vi "BuildHWI.vi"(8 "error in (no error)":errorcluster, 10 "Master Device in":refnum<class "Master Device.lvclass">, 11 "Advanced_DMD in":refnum<class "Advanced_DMD.lvclass">) -> (0 "error out":errorcluster, 2 "Master Device out":refnum<class "Master Device.lvclass">, 3 "Advanced_DMD out":refnum<class "Advanced_DMD.lvclass">)   [LabVIEW 2013, in "Advanced_DMD.lvclass"]
doc: "The previous subVI Prune.vi took the \"prepared\" private data and removed unnecessary points. Here in BuildHWI, one should turn the \"prepared\" data into a HWI that can be programmed to the physical device.\n (1) Flatten the data structure and put in normal time order"
uses:
  Advanced_DMD.lvclass
  Master Device/Master Device.lvclass
  Advanced_DMD.lvclass/Advanced_DMD.ctl
panel:
  out "appended path":path
  out "matlab command":string
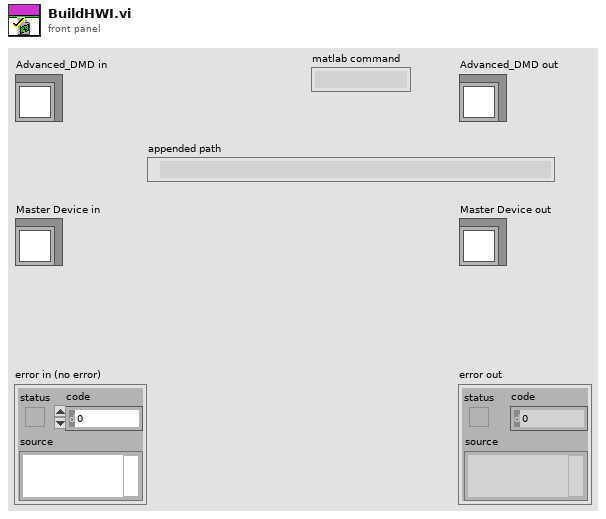
[diagram p1: front panel]
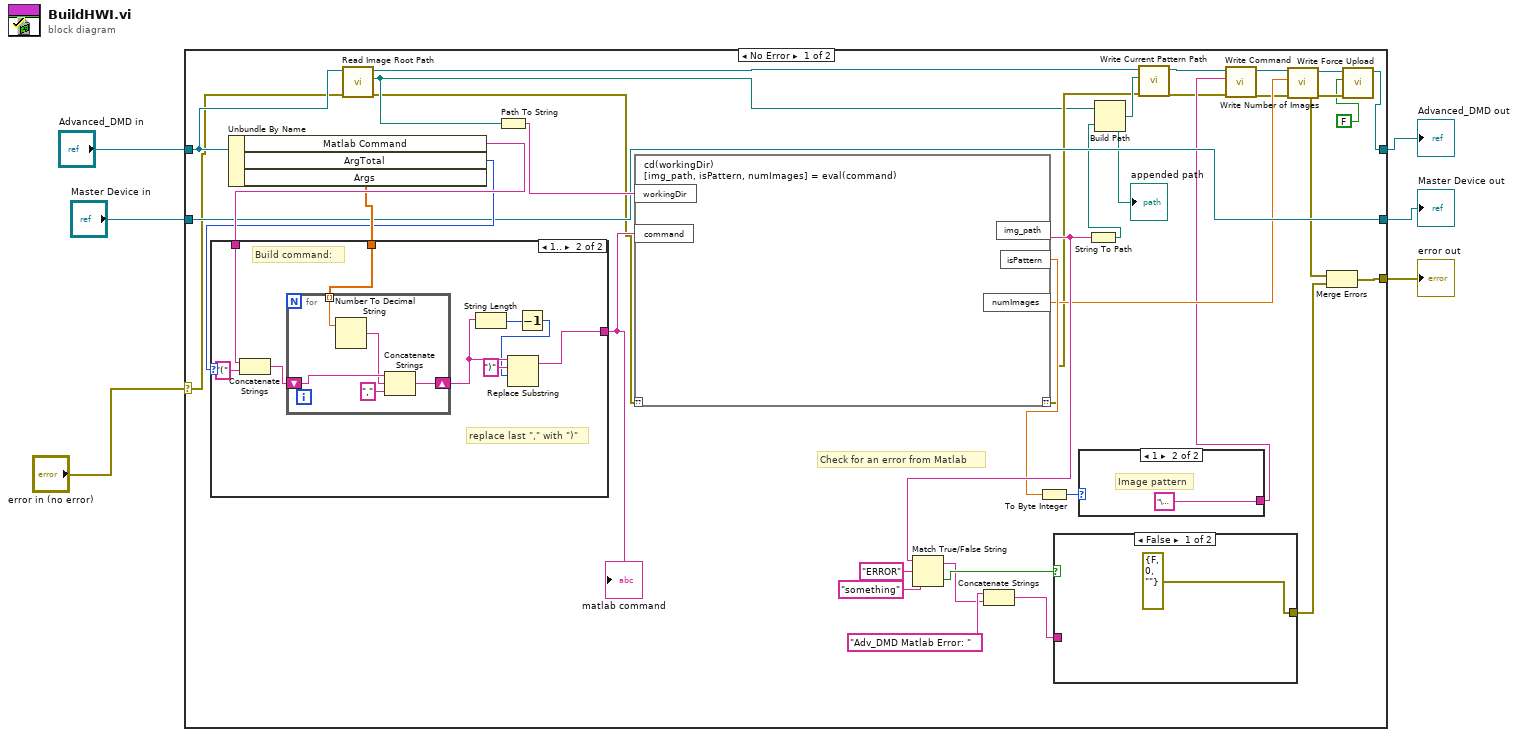
[diagram p0: block diagram]
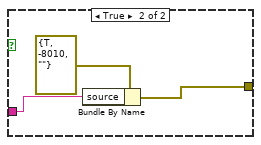
[diagram p2: hidden frame]
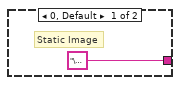
[diagram p3: hidden frame]
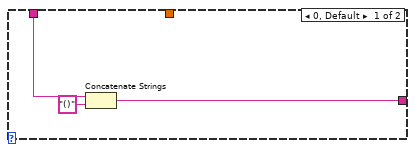
[diagram p4: hidden frame]
diagram:
  n1 = case shown="No Error" "error in (no error)" {
    selector: "error in (no error)" -> [w10 w66]
    tunnel: "Advanced_DMD in" -> [w11 w68]
    tunnel: [w20 w68] -> w4
    tunnel: [w37 w67] -> w3
    tunnel: "Master Device in" -> [w37 w67]
    tunnel: [w28 w66] -> w1
    frame No Error {
      # "Check for an error from Matlab"
      n2 = Unbundle By Name(w11) -> ("Matlab Command"=w41:string, "ArgTotal"=w39:u8, "Args"=w40:dbl[])
      n3 = case shown="1.." w39 {
        tunnel: w41 -> [w51 w59]
        tunnel: w40 -> [_ w57]
        tunnel: [w49 w52] -> w38
        frame 0, Default {
          n4 = Concatenate Strings(w51, "()" ("string")) -> (w49:string)
        }
        frame 1.. {
          # "replace last \",\" with \")\""
          # "Build command:"
          n5 = Concatenate Strings(w59, "(" ("string")) -> (w58:string)
          n6 = for {
            shift-right: [w61] -> w55
            shift-left: w58 -> [w65]
            tunnel: w57 -> [w64] mode=indexing
            n7 = Number To Decimal String(number=w64) -> (decimal integer string=w63:string)  [unwired: 1 in]
            n8 = Concatenate Strings(w65, w63, "," ("string")) -> (w61:string)
          }
          n9 = String Length(string=w55) -> (length=w56:i32)
          n10 = Decrement(x=w56) -> (x-1=w53:i32)
          n11 = Replace Substring(3:w53, 4:")" ("substring (\"\")"), 5:w55) -> (1:w52:string)  [unwired: 1 in, 1 out]
        }
      }
      "matlab command" <- w38
      n12 = call-dynamic "Read Image Root Path.vi"("error in (no error)"=w10, "DMD in"=w11) -> ("error out"=w8:errorcluster, "Image Root Path"=w9:path, "DMD out"=w7:refnum<class "Advanced_DMD.lvclass">)  [unwired: 7 in]
      n13 = Path To String(path=w9) -> (string=w42:string)
      n14 = script code="cd(workingDir)\n[img_path, isPattern, numImages] = eval(command)"("??"=w8, "workingDir"=w42, "command"=w38) -> ("??"=w17:errorcluster, "img_path"=w33:string, "isPattern"=w26:dbl, "numImages"=w19:dbl)
      n15 = Match True/False String(2:"something" ("false string"), 3:"ERROR" ("true string"), 4:w33) -> (0:w34:bool, 1:w30:string)
      n16 = Concatenate Strings("Adv_DMD Matlab Error: " ("false string"), w30) -> (w29:string)
      n17 = To Byte Integer(number=w26) -> (8bit integer=w25:i8)
      n18 = case shown="False" w34 {
        tunnel: [errorcluster {"status"=FALSE, "code"=0, "source"=""} ("error out") w44] -> w27
        tunnel: w29 -> [_ w45]
        frame False {
        }
        frame True {
          n19 = Bundle By Name(cluster=errorcluster {"status"=TRUE, "code"=-8010, "source"=""} ("error out"), "source"=w45) -> (w44:errorcluster)
        }
      }
      n20 = case shown="1" w25 {
        tunnel: ["\u0000" "\u0004"] -> w18
        frame 0, Default {
          # "Static Image"
        }
        frame 1 {
          # "Image pattern"
        }
      }
      n21 = String To Path(string=w33) -> (path=w36:path)
      n22 = Build Path(base path=w9, name or relative path=w36) -> (appended path=w24:path)
      "appended path" <- w24
      n23 = call-dynamic "Write Current Pattern Path.vi"("error in (no error)"=w17, "Current Pattern Path"=w24, "DMD in"=w7) -> ("error out"=w16:errorcluster, "DMD out"=w23:refnum<class "Advanced_DMD.lvclass">)  [unwired: 7 in]
      n24 = call-dynamic "Write Command.vi"("error in (no error)"=w16, "Command"=w18, "DMD in"=w23) -> ("error out"=w15:errorcluster, "DMD out"=w22:refnum<class "Advanced_DMD.lvclass">)  [unwired: 7 in]
      n25 = call-dynamic "Write Number of Images.vi"("error in (no error)"=w15, "Number of Images"=w19, "DMD in"=w22) -> ("error out"=w14:errorcluster, "DMD out"=w21:refnum<class "Advanced_DMD.lvclass">)  [unwired: 7 in]
      n26 = call-dynamic "Write Force Upload.vi"("error in (no error)"=w14, "Force Upload"=FALSE, "DMD in"=w21) -> ("error out"=w13:errorcluster, "DMD out"=w20:refnum<class "Advanced_DMD.lvclass">)  [unwired: 7 in]
      n27 = Merge Errors(w13, w27) -> (w28:errorcluster)
    }
    frame Error {
    }
  }
  "error out" <- w1
  "Advanced_DMD out" <- w4
  "Master Device out" <- w3
